vi "Write to Text File (with Core and Type).vi"(0 "Core":i32, 2 "Filetype":enum16{"Hardware", "Parameter"}(ring), 7 "Database Filepath (xlsx)":path=path "C:/Users/jkreienh/Desktop/Preliminary Ballard Database Template.xlsx", 11 "Error (in)":errorcluster) -> (15 "Error (out)":errorcluster)   [LabVIEW 2017]
panel:
  in  "Text":string
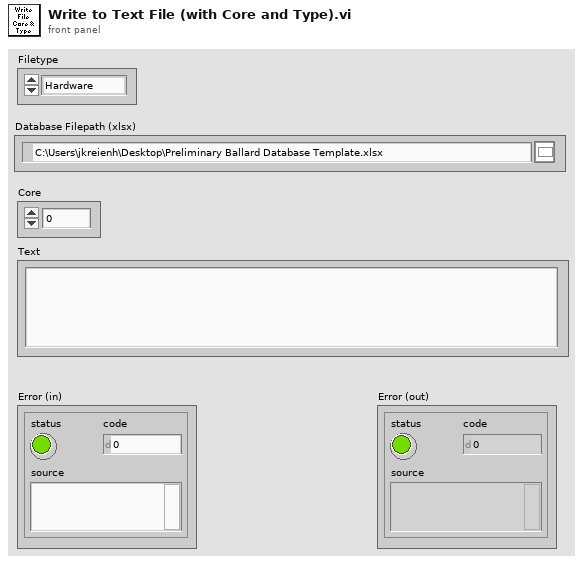
[diagram p1: front panel]
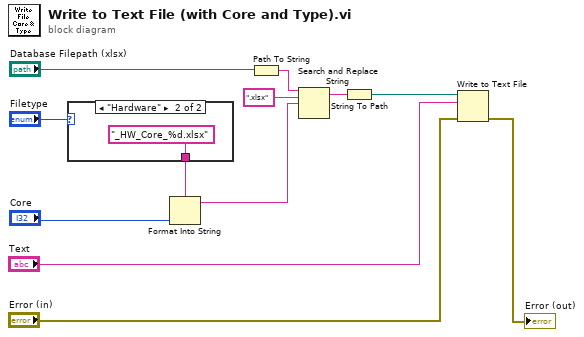
[diagram p0: block diagram]
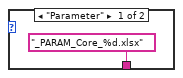
[diagram p2: hidden frame]
diagram:
  n1 = case shown="\"Hardware\"" "Filetype" {
    tunnel: ["_PARAM_Core_%d.xlsx" ("format string") "_HW_Core_%d.xlsx" ("format string")] -> w6
    frame "Parameter" {
    }
    frame "Hardware" {
    }
  }
  n2 = Format Into String(format string=w6, "Core") -> (resulting string=w9:string)  [unwired: 2 in, 1 out]
  n3 = Path To String(path="Database Filepath (xlsx)") -> (string=w11:string)
  n4 = Search and Replace String(input string=w11, search string=".xlsx", replace string=w9) -> (result string=w5:string)  [unwired: 5 in, 3 out]
  n5 = String To Path(string=w5) -> (path=w4:path)
  n6 = Write to Text File(file (use dialog)=w4, text="Text", error in="Error (in)") -> (error out=→"Error (out)":errorcluster)  [unwired: 1 in, 2 out]
